vi "CheckSN.vi"(6 "Slot":T1, 8 "error out":errorcluster, 11 "SN":string) -> (0 "错误输出":errorcluster, 3 "比对结果":bool)   [LabVIEW 2013]
uses:
  SystemCode/SysControl/Slot.ctl
panel:
  out "提示":string
  out "当前SN":string
  in  "扫描SN":string
  in  "停止":bool
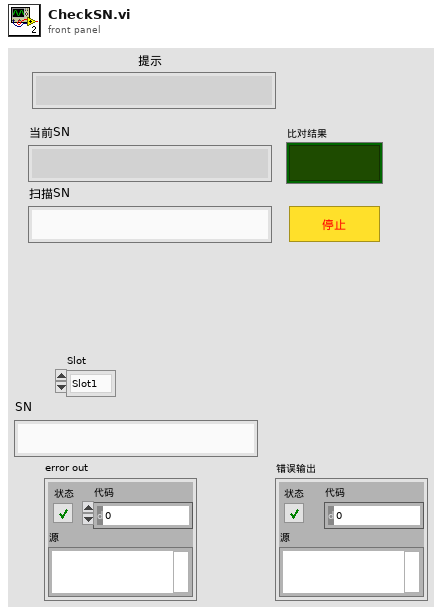
[diagram p1: front panel]
types:
  T1 = typedef "Slot.ctl" = enum16{"Slot1", "Slot2", "Slot3", "Slot4"}
  T2 = typedef "LVRectTypeDef.ctl" = cluster{"Left":i16, "Top":i16, "Right":i16, "Bottom":i16}
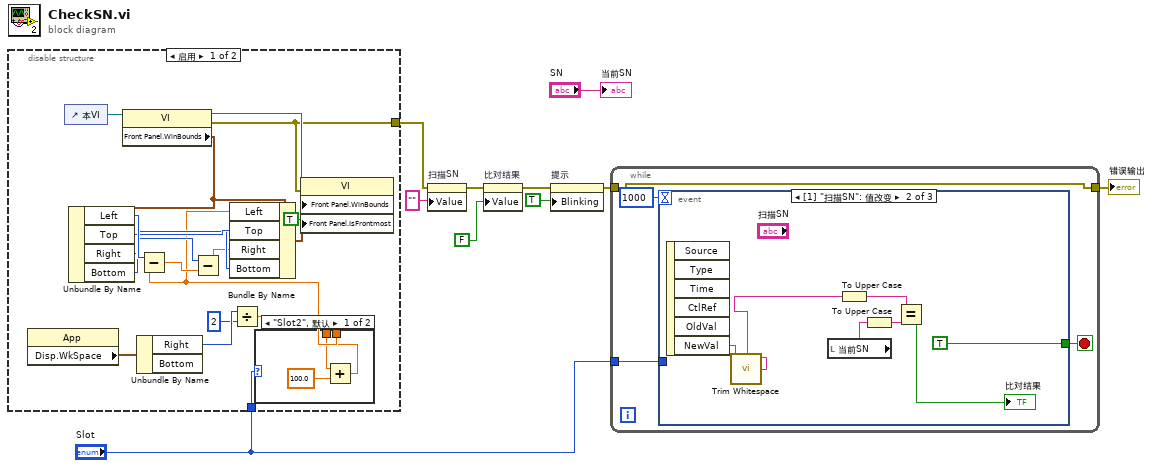
[diagram p0: block diagram]
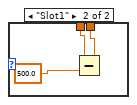
[diagram p2: hidden frame]
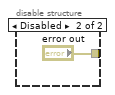
[diagram p3: hidden frame]
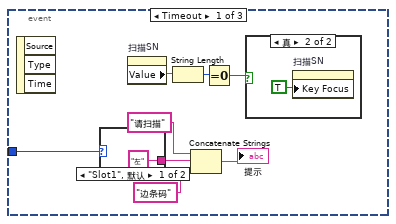
[diagram p4: hidden frame]
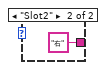
[diagram p5: hidden frame]
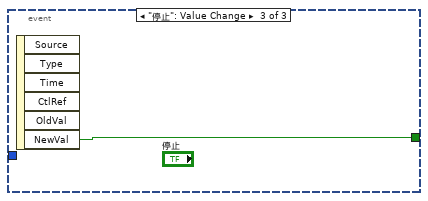
[diagram p7: hidden frame]
diagram:
  n1 = disable-structure shown="启用" {
    disable-tunnel: [w16 "error out"] -> w10
    disable-tunnel: "Slot" -> [w11 _]
    frame Enabled {
      n2 = property class="App"() -> ("Disp.WkSpace"=w25:T2)  [unwired: 2 in, 2 out]
      n3 = control-ref of="本VI"() -> (w28:refnum<vi>)
      n4 = property class="VI"(reference=w28) -> (reference out=w27:refnum<vi>, error out=w16:errorcluster, "Front Panel.WinBounds"=w23:T2)  [unwired: 1 in]
      n5 = Unbundle By Name(w23) -> ("Left"=w22:i16, "Top"=w21:i16, "Right"=w19:i16, "Bottom"=w20:i16)
      n6 = Unbundle By Name(w25) -> ("Right"=w15:i16)  [unwired: 1 out]
      n7 = Divide(x=w15, y=i16 2) -> (x/y=w13:dbl)
      n8 = case shown="\"Slot2\", 默认" w11 {
        tunnel: w13 -> [w31 w34]
        tunnel: [w29 w32] -> w12
        frame "Slot2", Default {
          n9 = Add(x=w31, y=100.0) -> (x+y=w29:dbl)
        }
        frame "Slot1" {
          n10 = Subtract(x=w34, y=500.0) -> (x-y=w32:dbl)
        }
      }
      n11 = Subtract(x=w22, y=w12) -> (x-y=w18:dbl)
      n12 = Subtract(x=w19, y=w18) -> (x-y=w17:dbl)
      n13 = Bundle By Name(cluster=w23, "Left"=w12, "Top"=w21, "Right"=w17, "Bottom"=w20) -> (w26:T2)
      n14 = property class="VI"(reference=w27, error in=w16, "Front Panel.WinBounds"=w26, "Front Panel.IsFrontmost"=TRUE ("前面板窗口:可调整大小")) -> ()  [unwired: 2 out]
    }
    frame Disabled {
    }
  }
  n15 = property on="扫描SN" class="Str"(error in=w10, "Value"="" ("扫描SN")) -> (error out=w5:errorcluster)  [unwired: 1 in, 1 out]
  n16 = property on="比对结果" class="Bool (严格)"(error in=w5, "Value"=FALSE ("比对结果")) -> (error out=w4:errorcluster)  [unwired: 1 in, 1 out]
  n17 = property on="提示" class="Str"(error in=w4, "Blinking"=TRUE ("闪烁")) -> (error out=w8:errorcluster)  [unwired: 1 in, 1 out]
  n18 = while {
    tunnel: w8 -> [w37]
    tunnel: [w37] -> w3
    tunnel: "Slot" -> [w36]
    stop <- w39 stop-if-true
    n19 = event shown="[1] \"扫描SN\": 值改变" {
      selector: _ -> [_ _ _]
      dyn-events: _ -> [_ _ _]
      timeout: 1000 -> [_ _ _]
      tunnel: [_ TRUE w58] -> w39
      tunnel: w36 -> [w40 _ _]
      event Timeout {
        n20 = event-data() -> ()  [unwired: 1 in, 3 out]
        n21 = case shown="\"Slot1\", 默认" w40 {
          tunnel: ["左" ("字符串") "右" ("字符串")] -> w41
          frame "Slot1", Default {
          }
          frame "Slot2" {
          }
        }
        n22 = property on="扫描SN" class="Str"() -> ("Value"=w47:string)  [unwired: 2 in, 2 out]
        n23 = String Length(string=w47) -> (length=w46:i32)
        n24 = Concatenate Strings("请扫描" ("字符串"), w41, "边条码" ("字符串")) -> (→"提示":string)
        n25 = Equal To 0?(x=w46) -> (x = 0?=w45:bool)
        n26 = case shown="真" w45 {
          frame False {
          }
          frame True {
            n27 = property on="扫描SN" class="Str"("Key Focus"=TRUE ("键选中")) -> ()  [unwired: 2 in, 2 out]
          }
        }
      }
      event "扫描SN": Value Change {
        n28 = event-data() -> ("NewVal"=w55:string)  [unwired: 1 in, 5 out]
        n29 = call <vilib>:"Trim Whitespace.vi"("string"=w55) -> ("trimmed string"=w54:string)  [unwired: 1 in]
        n30 = local read "当前SN"() -> (w51:string)
        n31 = To Upper Case(1:w54) -> (0:w52:string)
        n32 = To Upper Case(1:w51) -> (0:w53:string)
        n33 = Equal?(x=w52, y=w53) -> (x = y?=→"比对结果":bool)
      }
      event "停止": Value Change {
        n34 = event-data() -> ("NewVal"=w58:bool)  [unwired: 1 in, 5 out]
      }
    }
  }
  "错误输出" <- w3
  "当前SN" <- "SN"
